vi "Get Object Data.vi"(6 "Version ID":string, 8 "error in (no error)":errorcluster, 9 "Request Parameters":T2, 10 "Object Key":string, 11 "Bucket in":refnum<class "Bucket.lvclass">) -> (0 "error out":errorcluster, 1 "GetObjectResult":T1, 2 "Object Data":string, 3 "Bucket out":refnum<class "Bucket.lvclass">)   [LabVIEW 2015, in "NI_AWS_S3.lvlib" / "Bucket.lvclass"]
uses:
  Bucket.lvclass
  GET Object Request Parameters.ctl
  Core/Request Range.ctl
  GET Object Result Parameters.ctl
  Core/HTTP Request/Request Options.ctl
  Core/HTTP Request/Name Value Pair.ctl
  Core/HTTP Request/Region handling.ctl
  Core/HTTP Request/URL formatting.ctl
  Bucket.lvclass/Bucket.ctl
  Read Name.vi
  Core/HTTP Request/HTTP Request.lvclass
  Object/Object.lvclass
  NI_AWS_S3.lvlib
  Core/NI_AWS_Core.lvlib
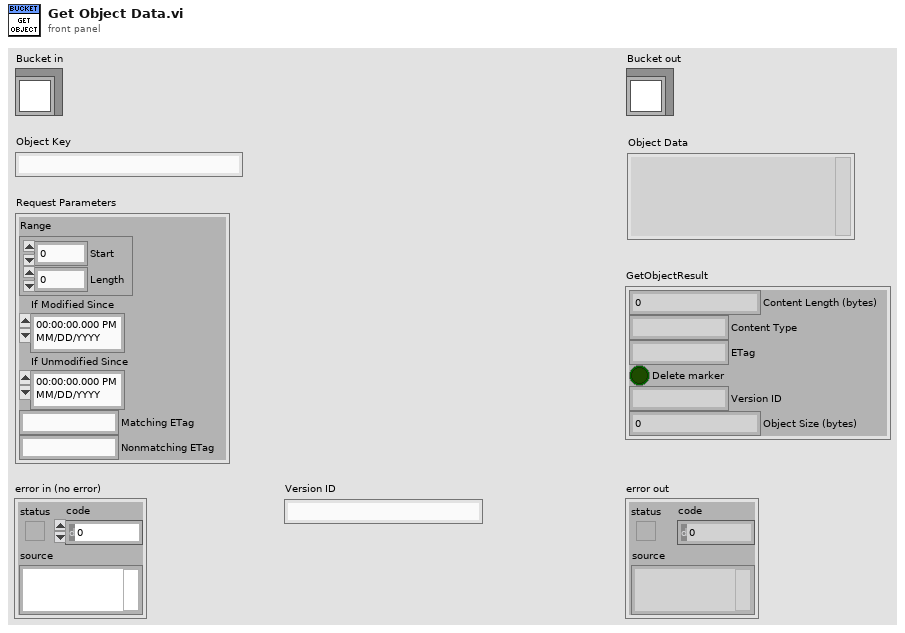
[diagram p1: front panel]
types:
  T1 = typedef "NI_AWS_S3.lvlib/GET Object Result Parameters.ctl" = cluster{"Content Length (bytes)":u64, "Content Type":string, "ETag":string, "Delete marker":bool, "Version ID":string, "Object Size (bytes)":u64}
  T2 = typedef "NI_AWS_S3.lvlib/GET Object Request Parameters.ctl" = cluster{"Range":T3, "If Modified Since":timestamp, "If Unmodified Since":timestamp, "Matching ETag":string, "Nonmatching ETag":string}
  T3 = typedef "NI_AWS_Core.lvlib/Request Range.ctl" = cluster{"Start":i64, "Length":i64}
  T4 = typedef "NI_AWS_Core.lvlib/HTTP Request.lvclass/Region handling.ctl" = enum16{"use region everywhere", "use region (authentication only)", "use region (URL only)", "ignore region everwhere"}
  T5 = typedef "NI_AWS_Core.lvlib/HTTP Request.lvclass/Request Options.ctl" = cluster{"request headers":T6[], "request parameters":T6[], "request body":string, "region handling":T4, "URL formatting":T7}
  T6 = typedef "NI_AWS_Core.lvlib/HTTP Request.lvclass/Name Value Pair.ctl" = cluster{"name":string, "value":string}
  T7 = typedef "NI_AWS_Core.lvlib/HTTP Request.lvclass/URL formatting.ctl" = enum16{"region-", "region."}
  T8 = typedef "NI_AWS_Core.lvlib/HTTP Request.lvclass/Response.ctl" = cluster{"Headers":string, "Body":string}
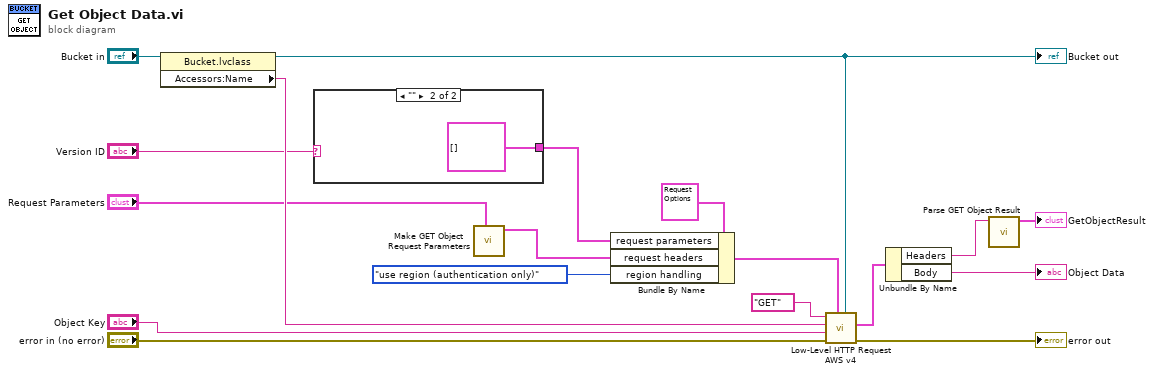
[diagram p0: block diagram]
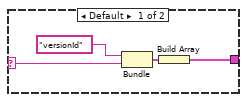
[diagram p2: hidden frame]
diagram:
  n1 = property class="Bucket.lvclass"(reference="Bucket in") -> (reference out=w12:refnum<class "Bucket.lvclass">, "Accessors:Name"=w15:string)  [unwired: 1 in, 1 out]
  "Bucket out" <- w12
  n2 = case shown="\"\"" "Version ID" {
    selector: "Version ID" -> [w19 _]
    tunnel: [w20 T6[] [] ("request parameters")] -> w8
    frame Default {
      n3 = Bundle("versionId", w19) -> (w21:cluster{string, string})  [unwired: 1 in]
      n4 = Build Array(w21) -> (w20:cluster{string, string}[])
    }
    frame "" {
    }
  }
  n5 = call "Make GET Object Request Parameters.vi"("GET Object Request Parameters"="Request Parameters") -> ("HTTP Headers"=w5:T6[])  [unwired: 9 in, 1 out]
  n6 = Bundle By Name(cluster=T5 {"request headers"=[], "request parameters"=[], "request body"="", "region handling"=enum."use region everywhere", "URL formatting"=enum."region."} ("Request Options"), "request parameters"=w8, "request headers"=w5, "region handling"=Region_handling."use region (authentication only)") -> (w16:T5)
  n7 = call "Low-Level HTTP Request AWS v4.vi"("AWS Core"=w12, "Request Options"=w16, "error in (no error)"="error in (no error)", "URL Suffix"="Object Key", "URL Prefix"=w15, "HTTP-Verb"="GET") -> ("error out"=→"error out":errorcluster, "Response"=w4:T8)  [unwired: 3 in, 1 out]
  n8 = Unbundle By Name(w4) -> ("Headers"=w2:string, "Body"=→"Object Data":string)
  n9 = call "Parse GET Object Result.vi"("Response header"=w2) -> ("GetObjectResult"=→"GetObjectResult":T1)  [unwired: 9 in, 1 out]
